vi "ITC4005_Set Temp+Stab time.vi"(8 "error in":errorcluster, 9 "Stabilization Time (s)":i32=120, 10 "TEC Temperature Setpoint (20.0)":dbl=25.0, 11 "ITC4005 handle in":refnum<visa-resource-name>="USB0::0x1313::0x804A::M00320668::INSTR" caption="instrument handle out") -> (0 "error out":errorcluster, 1 "At temp":bool=TRUE, 2 "Actual temperature":dbl=25.0067997 caption="Temperature", 3 "instrument handle out":refnum<visa-resource-name>="USB0::0x1313::0x804A::M00320668::INSTR")   [LabVIEW 2019]
panel:
  out "Stab Time":i32=13
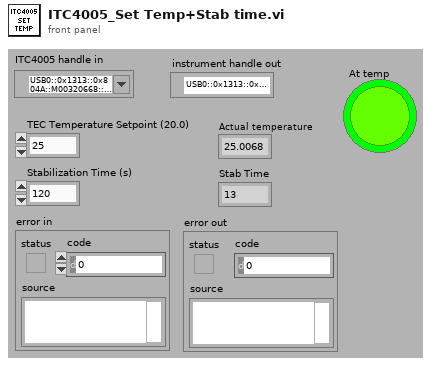
[diagram p1: front panel]
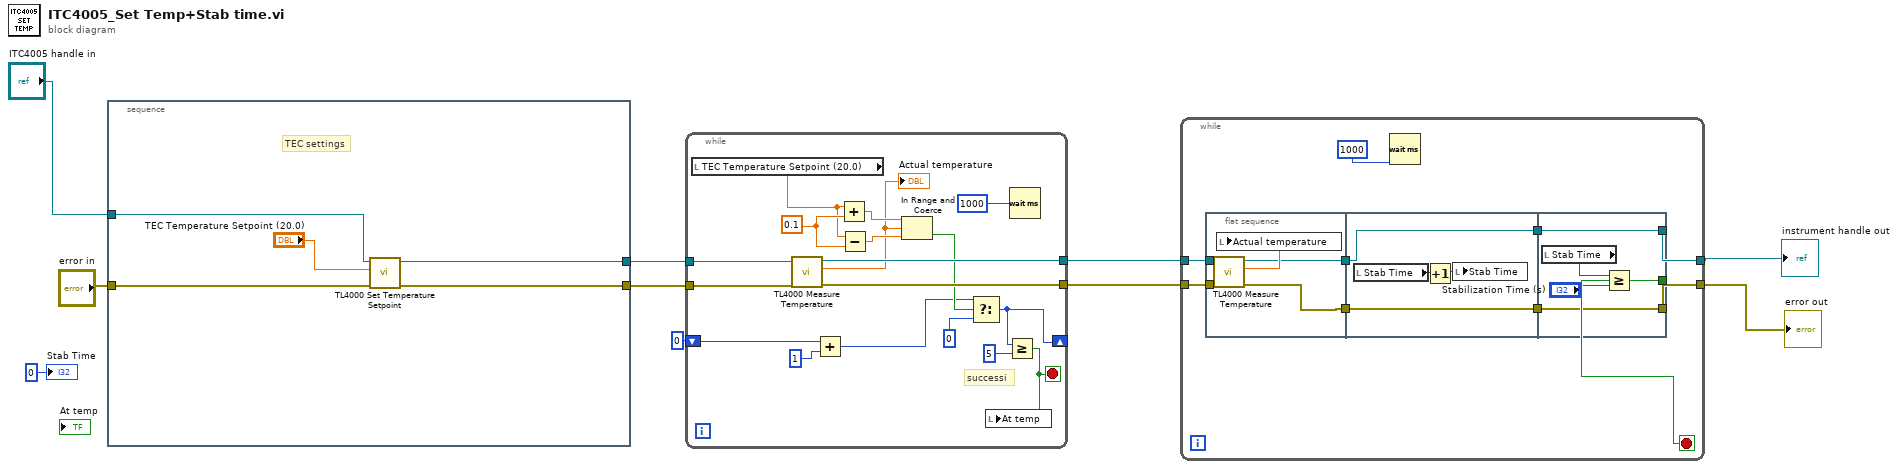
[diagram p0: block diagram]
diagram:
  n1 = stacked-sequence {
    tunnel: "error in" -> [w15]
    tunnel: [w14] -> w8
    tunnel: [w13] -> w7
    tunnel: "ITC4005 handle in" -> [w11]
    frame #0 {
      # "TEC settings"
      n2 = call <instrlib>:"TL4000 Set Temperature Setpoint.vi"("error in (no error)"=w15, "Temperature Setpoint (25.0)"="TEC Temperature Setpoint (20.0)", "instrument handle"=w11) -> ("error out"=w14:errorcluster, "instrument handle out"=w13:refnum<visa-resource-name>)  [unwired: 7 in]
    }
  }
  n3 = while {
    tunnel: w8 -> [w32]
    tunnel: w7 -> [w33]
    tunnel: [w31] -> w6
    tunnel: [w30] -> w5
    shift-right: [w23] -> _
    shift-left: 0 -> [w26]
    stop <- w16 stop-if-true
    w20 = 0.1 ("y")
    # "successi"
    n4 = local read "TEC Temperature Setpoint (20.0)"() -> (w17:dbl)
    n5 = call <instrlib>:"TL4000 Measure Temperature.vi"("error in (no error)"=w32, "instrument handle"=w33) -> ("error out"=w31:errorcluster, "Temperature"=w19:dbl, "instrument handle out"=w30:refnum<visa-resource-name>)  [unwired: 7 in]
    "Actual temperature" <- w19
    n6 = Add(x=w26, y=1) -> (x+y=w24:i32)
    n7 = Add(x=w17, y=w20) -> (x+y=w28:dbl)
    n8 = Subtract(x=w17, y=w20) -> (x-y=w29:dbl)
    n9 = In Range and Coerce(upper limit=w28, x=w19, lower limit=w29) -> (In Range?=w27:bool)  [unwired: 1 out]
    n10 = Select(t=w24, s=w27, f=0) -> (s? t:f=w23:i32)
    n11 = Greater Or Equal?(x=w23, y=5) -> (x >= y?=w16:bool)
    n12 = local write "At temp"(w16) -> ()
    n13 = Wait (ms)(milliseconds to wait=u32 1000) -> ()  [unwired: 1 out]
  }
  n14 = while {
    tunnel: w6 -> [w41]
    tunnel: w5 -> [w40]
    tunnel: [w34] -> w4
    tunnel: [w37] -> w3
    stop <- w42 stop-if-true
    n15 = flat-sequence {
      tunnel: w41 -> [w48]
      tunnel: w40 -> [w47]
      tunnel: [w45] -> w39
      tunnel: [w44] -> w36
      tunnel: w39 -> [w50]
      tunnel: [w50] -> w38
      tunnel: w36 -> [w49]
      tunnel: [w49] -> w35
      tunnel: [w55] -> w42
      tunnel: w38 -> [w54]
      tunnel: [w54] -> w37
      tunnel: w35 -> [w53]
      tunnel: [w53] -> w34
      frame #0 {
        n16 = call <instrlib>:"TL4000 Measure Temperature.vi"("error in (no error)"=w48, "instrument handle"=w47) -> ("error out"=w45:errorcluster, "Temperature"=w46:dbl, "instrument handle out"=w44:refnum<visa-resource-name>)  [unwired: 7 in]
        n17 = local write "Actual temperature"(w46) -> ()
      }
      frame #1 {
        n18 = local read "Stab Time"() -> (w52:i32)
        n19 = Increment(x=w52) -> (x+1=w51:i32)
        n20 = local write "Stab Time"(w51) -> ()
      }
      frame #2 {
        n21 = local read "Stab Time"() -> (w56:i32)
        n22 = Greater Or Equal?(x=w56, y="Stabilization Time (s)") -> (x >= y?=w55:bool)
      }
    }
    n23 = Wait (ms)(milliseconds to wait=u32 1000) -> ()  [unwired: 1 out]
  }
  "error out" <- w3
  "instrument handle out" <- w4
  "Stab Time" <- 0 ("Stab Time")
